vi "API_Set Operational Configuration.vi"(8 "error in (no error)":errorcluster, 10 "Tool OpCfg Params":T1={"Use Tool Cfg"=FALSE, "Use Tool Cal"=FALSE, "Fake Data?"=FALSE, "Mode"=-2, "Array Subset Length"=30, "nArrays to Read"=2, "Full Array Read Length"=500, "nSubarrays/Sensor"=0}) -> (0 "error out":errorcluster)   [LabVIEW 2015, in "Tool Module.lvlib"]
doc: "Sets the parameters in the ToolMgr: Operation Config Cluster."
uses:
  Tool Module.lvlib
  Tool Config/_Tool Operation Config Cluster--typedef.ctl
  Tool Config/Tool Cfg.lvlib
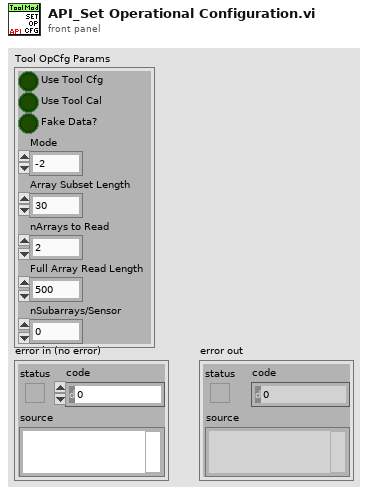
[diagram p1: front panel]
types:
  T1 = typedef "Tool Cfg.lvlib/_Tool Operation Config Cluster--typedef.ctl" = cluster{"Use Tool Cfg":bool, "Use Tool Cal":bool, "Fake Data?":bool, "Mode":i16, "Array Subset Length":i16, "nArrays to Read":i16, "Full Array Read Length":i16, "nSubarrays/Sensor":i16}
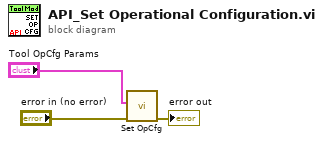
[diagram p0: block diagram]
diagram:
  n1 = call "Set OpCfg.vi"("error in (no error)"="error in (no error)", "Tool OpCfg Params"="Tool OpCfg Params") -> ("error out"=→"error out":errorcluster)  [unwired: 9 in]
